vi "GUI_CH1_Comm_Stream.vi"() -> ()   [LabVIEW 2018]
uses:
  Stream/Stream.lvclass
  RxTx/RxTx.lvclass
  Stream/Stream.lvclass/Stream.ctl
panel:
  in  "IP: 2":string="localhost"
  in  "RxTx.lvclass":refnum<class "RxTx.lvclass">
  in  "Stream.lvclass":refnum<class "Stream.lvclass">
  in  "RxTx.lvclass 2":refnum<class "RxTx.lvclass">
  in  "Stream.lvclass 2":refnum<class "Stream.lvclass">
  in  "Channel:":u16=1
  in  "IP:":string="localhost"
  # "Channel 1 Stream Communication"
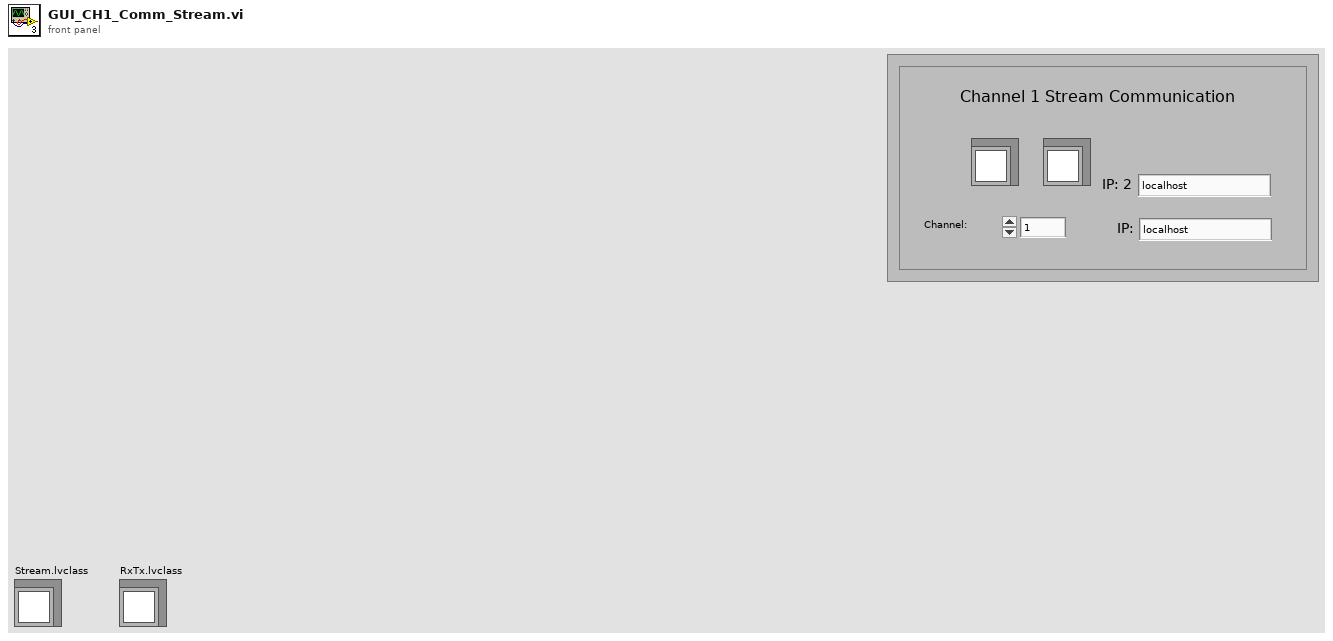
[diagram p1: front panel]
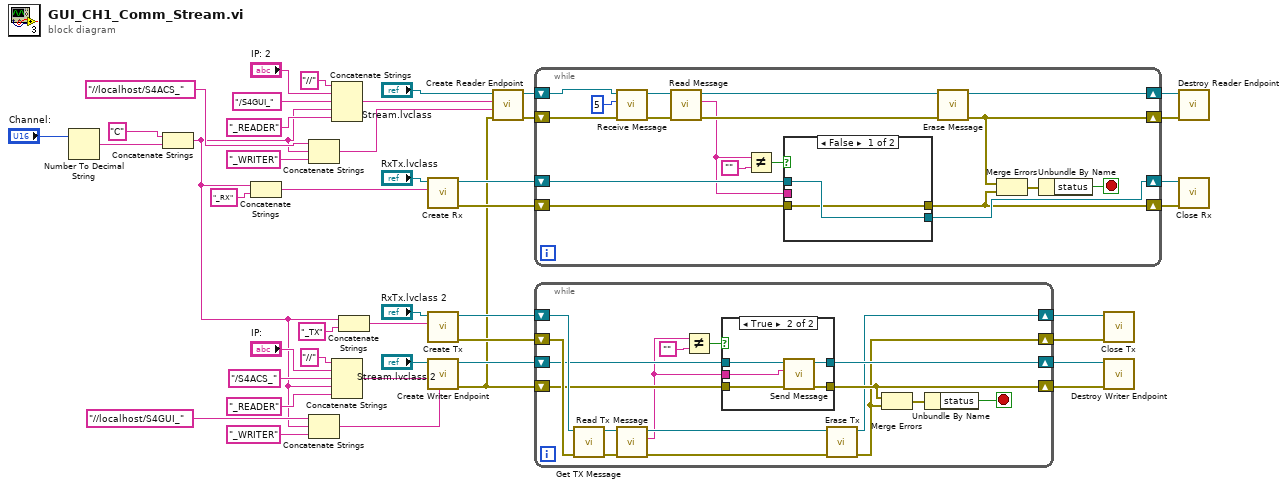
[diagram p0: block diagram]
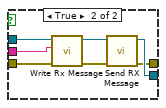
[diagram p2: hidden frame]
diagram:
  n1 = Number To Decimal String(number="Channel:") -> (decimal integer string=w15:string)  [unwired: 1 in]
  n2 = Concatenate Strings("C", w15) -> (w1:string)
  n3 = Concatenate Strings(w1, "_RX" ("Reader Name")) -> (w4:string)
  n4 = Concatenate Strings("//localhost/S4ACS_" ("reader name"), w1, "_WRITER" ("reader name")) -> (w11:string)
  n5 = Concatenate Strings("//localhost/S4GUI_" ("reader name"), w1, "_WRITER" ("reader name")) -> (w29:string)
  n6 = Concatenate Strings("//" ("Reader Name"), "IP: 2", "/S4GUI_" ("Reader Name"), w1, "_READER" ("Reader Name")) -> (w9:string)
  n7 = Concatenate Strings("//" ("Reader Name"), "IP:", "/S4ACS_" ("Reader Name"), w1, "_READER" ("Reader Name")) -> (w27:string)
  n8 = Concatenate Strings(w1, "_TX" ("Reader Name")) -> (w32:string)
  n9 = call "Create Rx.vi"("Reader Name"=w4, "RxTx in"="RxTx.lvclass") -> ("error out"=w5:errorcluster, "RxTx out"=w6:refnum<class "RxTx.lvclass">)  [unwired: 8 in]
  n10 = call "Create Tx.vi"("Writer Name"=w32, "RxTx in"="RxTx.lvclass 2") -> ("error out"=w42:errorcluster, "RxTx out"=w43:refnum<class "RxTx.lvclass">)  [unwired: 8 in]
  n11 = call "Create Writer Endpoint.vi"("writer name"=w29, "reader name"=w27, "Stream in"="Stream.lvclass 2") -> ("error out"=w2:errorcluster, "Stream out"=w39:refnum<class "Stream.lvclass">)  [unwired: 7 in]
  n12 = call "Create Reader Endpoint.vi"("error in (no error)"=w2, "writer name"=w11, "reader name"=w9, "Stream in"="Stream.lvclass") -> ("error out"=w20:errorcluster, "Stream out"=w22:refnum<class "Stream.lvclass">)  [unwired: 6 in]
  n13 = while {
    shift-right: [w45] -> w19
    shift-left: w20 -> [w59]
    shift-right: [w48] -> w25
    shift-left: w22 -> [w60]
    shift-right: [w50] -> w23
    shift-left: w5 -> [w52]
    shift-right: [w51] -> w24
    shift-left: w6 -> [w53]
    stop <- w61 stop-if-true
    n14 = call "Receive Message.vi"("error in (no error)"=w59, "timeout ms"=5, "Stream in"=w60) -> ("error out"=w57:errorcluster, "Stream out"=w56:refnum<class "Stream.lvclass">)  [unwired: 7 in]
    n15 = call "Read Message.vi"("error in (no error)"=w57, "Stream in"=w56) -> ("error out"=w49:errorcluster, "Message"=w46:string, "Stream out"=w47:refnum<class "Stream.lvclass">)  [unwired: 7 in]
    n16 = Not Equal?(x=w46, y="") -> (x != y?=w55:bool)
    n17 = case shown="False" w55 {
      tunnel: w53 -> [w64 w71]
      tunnel: w52 -> [w63 w70]
      tunnel: [w64 w67] -> w51
      tunnel: [w63 w66] -> w50
      tunnel: w46 -> [_ w65]
      frame False {
      }
      frame True {
        n18 = call "Write Rx Message.vi"("error in (no error)"=w70, "Rx Message"=w65, "RxTx in"=w71) -> ("error out"=w69:errorcluster, "RxTx out"=w68:refnum<class "RxTx.lvclass">)  [unwired: 7 in]
        n19 = call "Send RX Message.vi"("error in (no error)"=w69, "RxTx in"=w68) -> ("error out"=w66:errorcluster, "RxTx out"=w67:refnum<class "RxTx.lvclass">)  [unwired: 8 in]
      }
    }
    n20 = call "Erase Message.vi"("error in (no error)"=w49, "Stream in"=w47) -> ("error out"=w45:errorcluster, "Stream out"=w48:refnum<class "Stream.lvclass">)  [unwired: 8 in]
    n21 = Merge Errors(w45, w50) -> (w62:errorcluster)
    n22 = Unbundle By Name(w62) -> ("status"=w61:bool)
  }
  n23 = while {
    shift-right: [w81] -> w37
    shift-left: w2 -> [w83]
    shift-right: [w82] -> w44
    shift-left: w39 -> [w84]
    shift-right: [w76] -> w40
    shift-left: w42 -> [w85]
    shift-right: [w78] -> w41
    shift-left: w43 -> [w86]
    stop <- w72 stop-if-true
    n24 = call "Get TX Message.vi"("error in (no error)"=w85, "RxTx in"=w86) -> ("error out"=w87:errorcluster, "RxTx out"=w74:refnum<class "RxTx.lvclass">)  [unwired: 8 in]
    n25 = call "Read Tx Message.vi"("error in (no error)"=w87, "RxTx in"=w74) -> ("error out"=w77:errorcluster, "Tx Message"=w73:string, "RxTx out"=w79:refnum<class "RxTx.lvclass">)  [unwired: 7 in]
    n26 = Not Equal?(x=w73, y="") -> (x != y?=w75:bool)
    n27 = case shown="True" w75 {
      tunnel: w84 -> [w90 w95]
      tunnel: w83 -> [w89 w94]
      tunnel: [w90 w93] -> w82
      tunnel: w73 -> [_ w92]
      tunnel: [w89 w91] -> w81
      frame False {
      }
      frame True {
        n28 = call "Send Message.vi"("error in (no error)"=w94, "Message"=w92, "Stream in"=w95) -> ("error out"=w91:errorcluster, "Stream out"=w93:refnum<class "Stream.lvclass">)  [unwired: 7 in]
      }
    }
    n29 = call "Erase Tx.vi"("error in (no error)"=w77, "RxTx in"=w79) -> ("error out"=w76:errorcluster, "RxTx out"=w78:refnum<class "RxTx.lvclass">)  [unwired: 8 in]
    n30 = Merge Errors(w81, w76) -> (w88:errorcluster)
    n31 = Unbundle By Name(w88) -> ("status"=w72:bool)
  }
  n32 = call "Close Tx.vi"("error in (no error)"=w40, "RxTx in"=w41) -> ()  [unwired: 8 in, 2 out]
  n33 = call "Destroy Writer Endpoint.vi"("error in (no error)"=w37, "Stream in"=w44) -> ()  [unwired: 8 in, 2 out]
  n34 = call "Destroy Reader Endpoint.vi"("error in (no error)"=w19, "Stream in"=w25) -> ()  [unwired: 8 in, 2 out]
  n35 = call "Close Rx.vi"("error in (no error)"=w23, "RxTx in"=w24) -> ()  [unwired: 8 in, 2 out]
